vi "onAddHeader.vi"(8 "error in":errorcluster, 9 "value":string, 10 "header":string, 11 "advanced-http-client in":refnum<class "advanced-http-client.lvclass">) -> (0 "error out":errorcluster, 3 "advanced-http-client out":refnum<class "advanced-http-client.lvclass">)   [LabVIEW 2020, in "HttpClient.NiAdvanced.lvlib" / "advanced-http-client.lvclass"]
uses:
  advanced-http-client.lvclass
  advanced-http-client.lvclass/advanced-http-client.ctl
  <vilib>/NI/Advanced HTTP Client/Session.lvclass
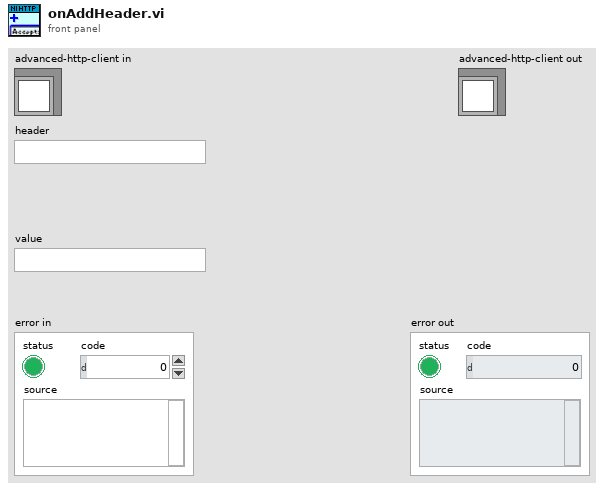
[diagram p1: front panel]
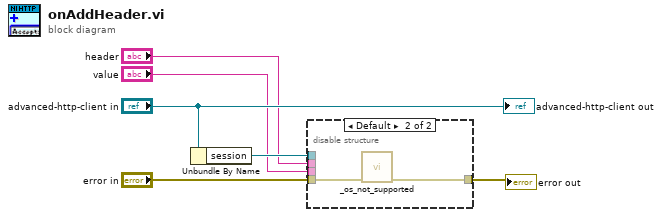
[diagram p0: block diagram]
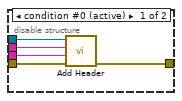
[diagram p2: hidden frame]
diagram:
  n1 = Unbundle By Name("advanced-http-client in") -> ("session"=w5:refnum<class "Session.lvclass">)
  n2 = disable-structure shown="Default" {
    disable-tunnel: w5 -> [w11 _]
    disable-tunnel: "header" -> [w10 _]
    disable-tunnel: "value" -> [w9 _]
    disable-tunnel: "error in" -> [w8 w13]
    disable-tunnel: [w7 w12] -> w1
    frame condition #0 (active) {
      n3 = call <vilib>:"Add Header.vi"("error in"=w8, "value"=w9, "header"=w10, "session in"=w11) -> ("error out"=w7:errorcluster)  [unwired: 6 in, 1 out]
    }
    frame condition #1 {
      n4 = call "_os_not_supported.vi"("error in (no error)"=w13) -> ("error out"=w12:errorcluster)  [unwired: 9 in, 1 out]
    }
  }
  "error out" <- w1
  "advanced-http-client out" <- "advanced-http-client in"
